vi "set_PulseWidth_subvi.vi"(0 "Pulsewidth":dbl, 1 "Combined Format? (False) in":bool, 5 "10-bit Addressing? (False) in":bool, 7 "No Stop? (False) in":bool, 9 "Aardvark Handle in":i32 min=0, 11 "error in (no error)":errorcluster, 12 "Address (0x50) in":u16=80 max=1023 format="%.0x") -> (2 "x1,25ns":u8[](array[numeric]) format="%.0x", 3 "Boolean array 4":bool[](array[boolean]), 4 "dup Aardvark Handle 2":i32, 6 "Num Bytes Written 3":u16, 8 "Status 3":i32, 10 "x 10ns 3":u8[](array[numeric]) format="%.0x", 14 "Boolean array 3":bool[](array[boolean]), 15 "error out":errorcluster)   [LabVIEW 2014]
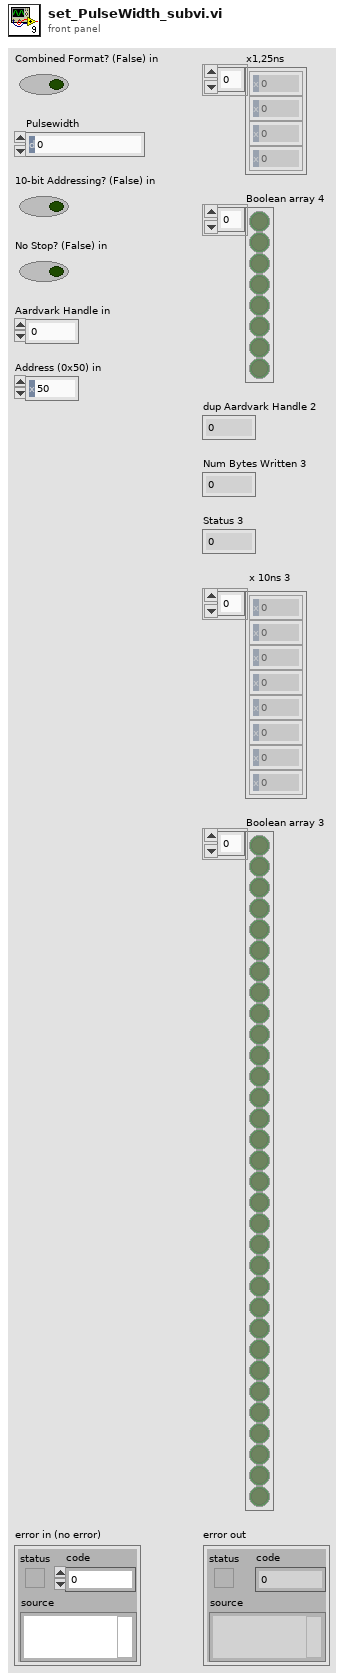
[diagram p1: front panel]
types:
  T1 = cluster{"unsigned byte array[0]":u8, "unsigned byte array[1]":u8, "unsigned byte array[2]":u8, "unsigned byte array[3]":u8, "unsigned byte array[4]":u8, "unsigned byte array[5]":u8, "unsigned byte array[6]":u8, "unsigned byte array[7]":u8, "unsigned byte array[8]":u8}
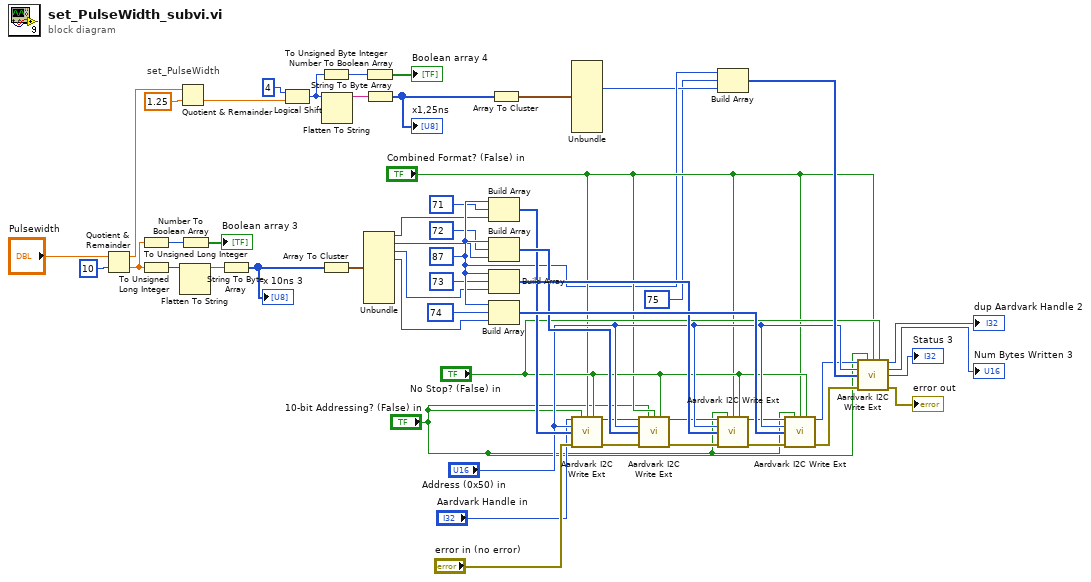
[diagram p0: block diagram]
diagram:
  w30 = u8 87
  # "set_PulseWidth"
  n1 = Quotient & Remainder(x="Pulsewidth", y=10) -> (x-y*floor(x/y)=w3:dbl, floor(x/y)=w14:dbl)
  n2 = To Unsigned Long Integer(number=w14) -> (unsigned 32bit integer=w7:u32)
  n3 = To Unsigned Long Integer(number=w14) -> (unsigned 32bit integer=w15:u32)
  n4 = Quotient & Remainder(x=w3, y=1.25) -> (floor(x/y)=w6:dbl)  [unwired: 1 out]
  n5 = Flatten To String(anything=w15) -> (data string=w9:string)  [unwired: 3 in, 2 out]
  n6 = Number To Boolean Array(number=w7) -> (Boolean array=→"Boolean array 3":bool[])
  n7 = String To Byte Array(string=w9) -> (unsigned byte array=w16:u8[])
  "x 10ns 3" <- w16
  n8 = Logical Shift(y=4, x=w6) -> (x << y=w13:u32)
  n9 = To Unsigned Byte Integer(number=w13) -> (unsigned 8bit integer=w11:u8)
  n10 = Array To Cluster(array=w16) -> (cluster=w17:T1)
  n11 = Flatten To String(anything=w13) -> (data string=w12:string)  [unwired: 3 in, 2 out]
  n12 = Unbundle(w17) -> ("unsigned byte array[0]"=w19:u8, "unsigned byte array[1]"=w24:u8, "unsigned byte array[2]"=w25:u8, "unsigned byte array[3]"=w26:u8)  [unwired: 5 out]
  n13 = Number To Boolean Array(number=w11) -> (Boolean array=→"Boolean array 4":bool[])
  n14 = String To Byte Array(string=w12) -> (unsigned byte array=w27:u8[])
  "x1,25ns" <- w27
  n15 = Build Array(w30, u16 71, w19) -> (w46:u16[])
  n16 = Build Array(w30, u16 72, w24) -> (w47:u16[])
  n17 = Build Array(w30, u16 73, w25) -> (w48:u16[])
  n18 = Build Array(w30, u16 74, w26) -> (w49:u16[])
  n19 = Array To Cluster(array=w27) -> (cluster=w28:T1)
  n20 = Unbundle(w28) -> ("unsigned byte array[3]"=w29:u8)  [unwired: 8 out]
  n21 = call <instrlib>:"Aardvark I2C Write Ext.vi"("Aardvark Handle"="Aardvark Handle in", "10-bit Addressing? (False)"="10-bit Addressing? (False) in", "Combined Format? (False)"="Combined Format? (False) in", "No Stop? (False)"="No Stop? (False) in", "Address (0x50)"="Address (0x50) in", "Data to Write"=w46, "error in (no error)"="error in (no error)") -> ("dup Aardvark Handle"=w33:i32, "error out"=w41:errorcluster)  [unwired: 5 in, 2 out]
  n22 = call <instrlib>:"Aardvark I2C Write Ext.vi"("Aardvark Handle"=w33, "10-bit Addressing? (False)"="10-bit Addressing? (False) in", "Combined Format? (False)"="Combined Format? (False) in", "No Stop? (False)"="No Stop? (False) in", "Address (0x50)"="Address (0x50) in", "Data to Write"=w47, "error in (no error)"=w41) -> ("dup Aardvark Handle"=w34:i32, "error out"=w42:errorcluster)  [unwired: 5 in, 2 out]
  n23 = Build Array(w30, u16 75, w29) -> (w50:u16[])
  n24 = call <instrlib>:"Aardvark I2C Write Ext.vi"("Aardvark Handle"=w34, "10-bit Addressing? (False)"="10-bit Addressing? (False) in", "Combined Format? (False)"="Combined Format? (False) in", "No Stop? (False)"="No Stop? (False) in", "Address (0x50)"="Address (0x50) in", "Data to Write"=w48, "error in (no error)"=w42) -> ("dup Aardvark Handle"=w35:i32, "error out"=w43:errorcluster)  [unwired: 5 in, 2 out]
  n25 = call <instrlib>:"Aardvark I2C Write Ext.vi"("Aardvark Handle"=w35, "10-bit Addressing? (False)"="10-bit Addressing? (False) in", "Combined Format? (False)"="Combined Format? (False) in", "No Stop? (False)"="No Stop? (False) in", "Address (0x50)"="Address (0x50) in", "Data to Write"=w49, "error in (no error)"=w43) -> ("dup Aardvark Handle"=w36:i32, "error out"=w44:errorcluster)  [unwired: 5 in, 2 out]
  n26 = call <instrlib>:"Aardvark I2C Write Ext.vi"("Aardvark Handle"=w36, "10-bit Addressing? (False)"="10-bit Addressing? (False) in", "Combined Format? (False)"="Combined Format? (False) in", "No Stop? (False)"="No Stop? (False) in", "Address (0x50)"="Address (0x50) in", "Data to Write"=w50, "error in (no error)"=w44) -> ("dup Aardvark Handle"=→"dup Aardvark Handle 2":i32, "Num Bytes Written"=→"Num Bytes Written 3":u16, "Status"=→"Status 3":i32, "error out"=→"error out":errorcluster)  [unwired: 5 in]
